vi "Flatten Warning.vi"(8 "Error In":errorcluster, 9 "UIP Name":string, 10 "Label.Text":string) -> (0 "Error Out":errorcluster)   [LabVIEW 2015, in "UIM.lvclass"]
uses:
  UIM.lvclass
  <vilib>/Utility/error.llb/Error Cluster From Error Code.vi
  <vilib>/ErrorRing/Error Ring.xnode
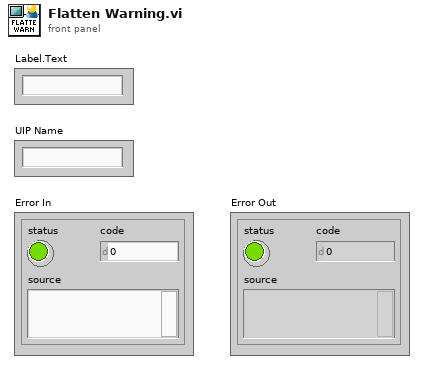
[diagram p1: front panel]
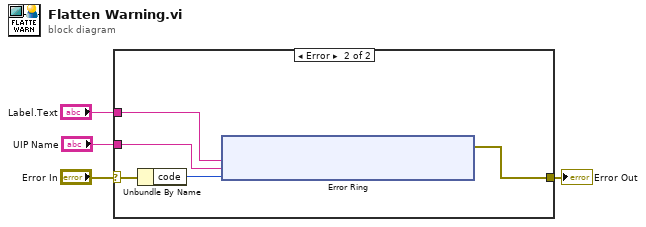
[diagram p0: block diagram]
diagram:
  n1 = case shown="Error" "Error In" {
    selector: "Error In" -> [w5 w10]
    tunnel: "Label.Text" -> [_ w9]
    tunnel: [w5 w6] -> w4
    tunnel: "UIP Name" -> [_ w8]
    frame No Error {
    }
    frame Error {
      n2 = Unbundle By Name(w10) -> ("code"=w7:i32)
      n3 = xnode "Error Ring"("parameter 0"=w9, "parameter 1"=w8, "parameter 2"=w7) -> ("error out"=w6:errorcluster)
    }
  }
  "Error Out" <- w4
